vi "getValue.vi"(8 "error in (no error)":errorcluster, 11 "type in":refnum<class "type.lvclass">) -> (0 "error out":errorcluster, 2 "value":variant, 3 "type out":refnum<class "type.lvclass">)   [LabVIEW 2015, in "type.lvclass"]
uses:
  type.lvclass
  type.lvclass/type.ctl
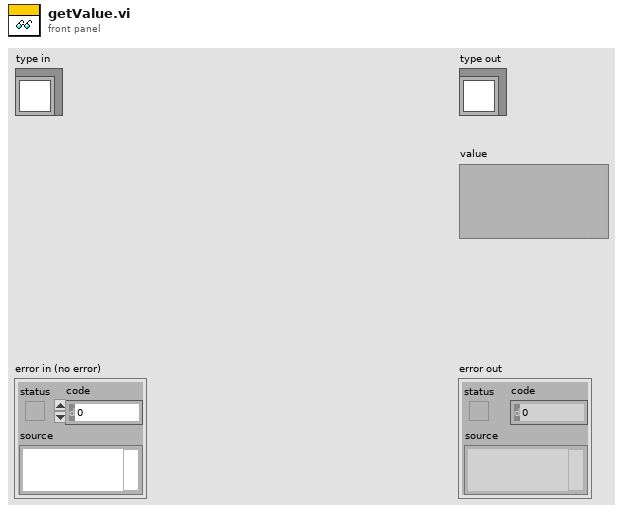
[diagram p1: front panel]
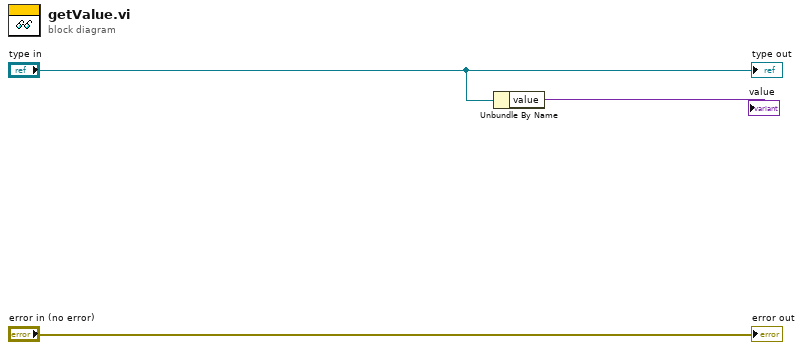
[diagram p0: block diagram]
diagram:
  n1 = Unbundle By Name("type in") -> ("value"=→"value":variant)
  "error out" <- "error in (no error)"
  "type out" <- "type in"
